vi "digital-Trigger.vi"(5 "trigger slope":u16(ring)=1 items=["Falling Edge", "Rising Edge"], 6 "signal in":dbl[](array[numeric])=[0.0], 8 "level":dbl=2.0, 9 "trigger in":dbl[](array[numeric])) -> (0 "signal out":dbl[](array[numeric]), 2 "trigger location":i32, 3 "trigger out":dbl[](array[numeric]))   [LabVIEW 2014]
doc: "André Romero - 2016\nandretec@ifsc.usp.br"
uses:
  <vilib>/measure/mamon.llb/Trigger Detection for 1 Channel.vi
  <vilib>/measure/NI_MAPro.lvlib
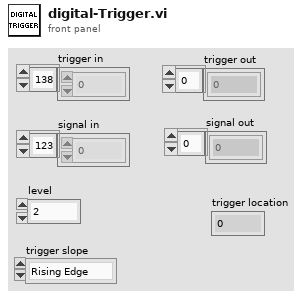
[diagram p1: front panel]
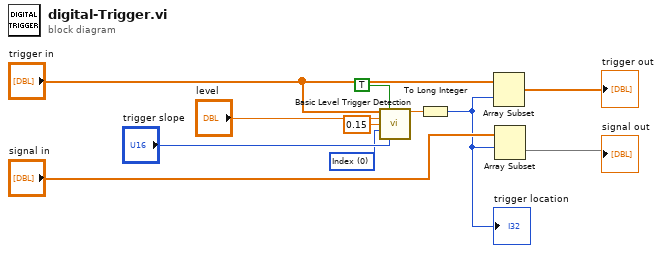
[diagram p0: block diagram]
diagram:
  w2 = u16 0 items=["Index", "Time"] ("location mode")
  n1 = call-poly <vilib>:"Basic Level Trigger Detection.vi"("signal in"="trigger in", "reset"=TRUE, "level"="level", "hysteresis"=0.15, "location mode"=w2, "trigger slope"="trigger slope") -> ("trigger location"=w11:dbl)  [unwired: 7 in, 2 out]
  n2 = To Long Integer(number=w11) -> (32bit integer=w1:i32)
  "trigger location" <- w1
  n3 = Array Subset "Array Subset"(array="trigger in", index=w1) -> (→"trigger out":dbl[])  [unwired: 1 in]
  n4 = Array Subset(array="signal in", index=w1) -> (→"signal out":dbl[])  [unwired: 1 in]
